vi "Module Type.vi"(11 "Data Logger BOOL Module in":refnum<class "Data Logger BOOL Module.lvclass">) -> (2 "Module Type":string)   [LabVIEW 2020, in "VolatusData.lvlib" / "Data Logger BOOL Module.lvclass"]
uses:
  Data Logger BOOL Module.lvclass
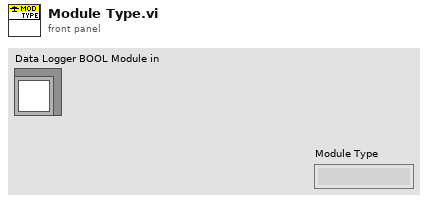
[diagram p1: front panel]
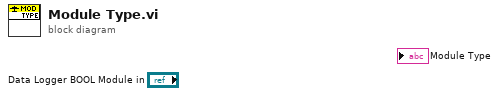
[diagram p0: block diagram]
diagram:
